vi "auto_test.vi"() -> ()   [LabVIEW 2019]
uses:
  auto_simple_straight.ctl
  <vilib>/Rock Robotics/Network Tables/NT Write Numeric Array.vi
  <vilib>/Rock Robotics/WPI/RobotDrive/WPI_RobotDriveArcadeDrive_Standard(NoSaturation).vi
  <vilib>/Rock Robotics/WPI/Solenoid/WPI_SolenoidValue.ctl
  <vilib>/Rock Robotics/WPI/Solenoid/WPI_SolenoidSetEnum.vi
  <vilib>/Rock Robotics/WPI/ThirdParty/Phoenix-LabVIEW/Motor Controller/Controls/CTRE_Phoenix_MotorControl_ControlMode.ctl
panel:
  out "Output Countdown\nTimer":dbl
  out "Motors and Solenoids On":bool
  out "Auto State":T1
  in  "Abort":bool
  in  "Intake Control":T2 items=["PercentOutput"=0, "Position"=1, "Velocity"=2, "Current"=3, "Follower"=5, "MotionProfile"=6, "MotionMagic"=7, "MotionProfileArc"=10, "Disabled"=15]
  in  "Output Control":T2 items=["PercentOutput"=0, "Position"=1, "Velocity"=2, "Current"=3, "Follower"=5, "MotionProfile"=6, "MotionMagic"=7, "MotionProfileArc"=10, "Disabled"=15]
  in  "Climber Control":T2 items=["PercentOutput"=0, "Position"=1, "Velocity"=2, "Current"=3, "Follower"=5, "MotionProfile"=6, "MotionMagic"=7, "MotionProfileArc"=10, "Disabled"=15]
  in  "Winch Control":T2 items=["PercentOutput"=0, "Position"=1, "Velocity"=2, "Current"=3, "Follower"=5, "MotionProfile"=6, "MotionMagic"=7, "MotionProfileArc"=10, "Disabled"=15]
  in  "Output Control 2":T2 items=["PercentOutput"=0, "Position"=1, "Velocity"=2, "Current"=3, "Follower"=5, "MotionProfile"=6, "MotionMagic"=7, "MotionProfileArc"=10, "Disabled"=15]
  in  "Intake Control":T2 items=["PercentOutput"=0, "Position"=1, "Velocity"=2, "Current"=3, "Follower"=5, "MotionProfile"=6, "MotionMagic"=7, "MotionProfileArc"=10, "Disabled"=15]
  in  "Climber Control":T2 items=["PercentOutput"=0, "Position"=1, "Velocity"=2, "Current"=3, "Follower"=5, "MotionProfile"=6, "MotionMagic"=7, "MotionProfileArc"=10, "Disabled"=15]
  in  "Winch Control":T2 items=["PercentOutput"=0, "Position"=1, "Velocity"=2, "Current"=3, "Follower"=5, "MotionProfile"=6, "MotionMagic"=7, "MotionProfileArc"=10, "Disabled"=15]
  in  "Output Control":T2 items=["PercentOutput"=0, "Position"=1, "Velocity"=2, "Current"=3, "Follower"=5, "MotionProfile"=6, "MotionMagic"=7, "MotionProfileArc"=10, "Disabled"=15]
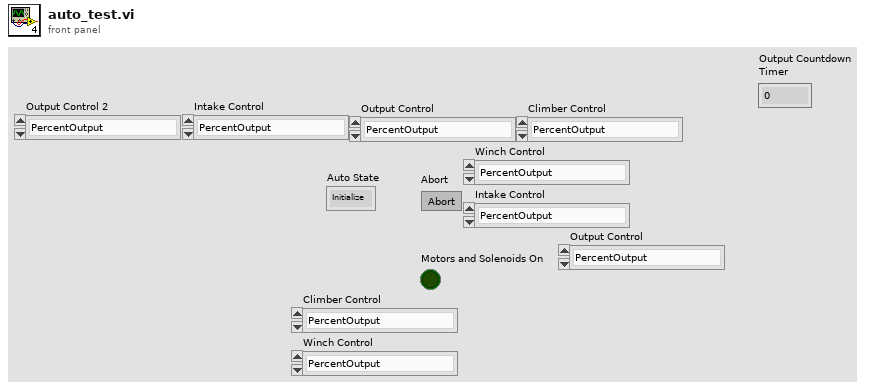
[diagram p1: front panel]
types:
  T1 = typedef "auto_simple_straight.ctl" = enum16{"Initialize", "Ready", "Move Forward", "Start Output Countdown", "Countdown", "Enable Output and Stop Drive", "Abort", "Motors Off"}
  T2 = typedef "CTRE_Phoenix_MotorControl_ControlMode.ctl" = u16
  T3 = typedef "WPI_SolenoidValue.ctl" = enum16{"Off", "On", "Forward", "Reverse"}
  T4 = typedef "WPI_RobotDriveDevRef.ctl" = cluster{"DevStatus":errorcluster, "Motors[]":T5[], "Square Inputs":bool, "Max Output":dbl}
  T5 = typedef "WPI_MotorControlDeviceRef.ctl" = cluster{"DeviceStatus":errorcluster, "Type":T6, "PWM":cluster{"PWM Channel":T7, "DeadBand":T8}, "CAN":cluster{"Device Number":u8, "SetOutput VI Ref":variant, "GetOutput VI Ref":variant, "Enable VI Ref":variant, "Disable VI Ref":variant, "Data":variant}, "Invert":bool, "DIO PWM":cluster{"PWM \"Enable\" Channel":T7, "DIOChannel":T9, "PWM Rate":dbl}}
  T6 = typedef "WPI_MotorControlType.ctl" = enum16{"PWM", "CAN", "DIO PWM"}
  T7 = typedef "FPGA_DIOPWMChannel.ctl" = enum8{"PWM 0", "PWM 1", "PWM 2", "PWM 3", "PWM 4", "PWM 5", "PWM 6", "PWM 7", "PWM 8", "PWM 9", "PWM MXP 0", "PWM MXP 1", "PWM MXP 2", "PWM MXP 3", "PWM MXP 4", "PWM MXP 5", "PWM MXP 6", "PWM MXP 7", "PWM MXP 8", "PWM MXP 9", "Invalid"}
  T8 = typedef "WPI_PWMDeadband.ctl" = cluster{"Name":string, "maxPositivePwm":i32, "minPositivePwm":i32, "centerPwm":i32, "maxNegativePwm":i32, "minNegativePwm":i32, "angularRange":u16}
  T9 = typedef "FPGA_DIOChannel.ctl" = enum8{"DIO 0", "DIO 1", "DIO 2", "DIO 3", "DIO 4", "DIO 5", "DIO 6", "DIO 7", "DIO 8", "DIO 9", "DIO MXP 0", "DIO MXP 1", "DIO MXP 2", "DIO MXP 3", "DIO MXP 4", "DIO MXP 5", "DIO MXP 6", "DIO MXP 7", "DIO MXP 8", "DIO MXP 9", "DIO MXP 10", "DIO MXP 11", "DIO MXP 12", "DIO MXP 13", "DIO MXP 14", "DIO MXP 15", "SPI Port CS1", "SPI Port CS2", "SPI Port CS3", "SPI Port MISO", "SPI Port MOSI", "Invalid"}
  T10 = typedef "WPI_SolenoidDevRef.ctl" = cluster{"DevStatus":errorcluster, "Pneumatics Control Module":u8, "Forward Solenoid Channel":T11, "Reverse Solenoid Channel":T11}
  T11 = typedef "WPI_SolenoidChannel.ctl" = enum8{"Solenoid 0", "Solenoid 1", "Solenoid 2", "Solenoid 3", "Solenoid 4", "Solenoid 5", "Solenoid 6", "Solenoid 7", "Invalid"}
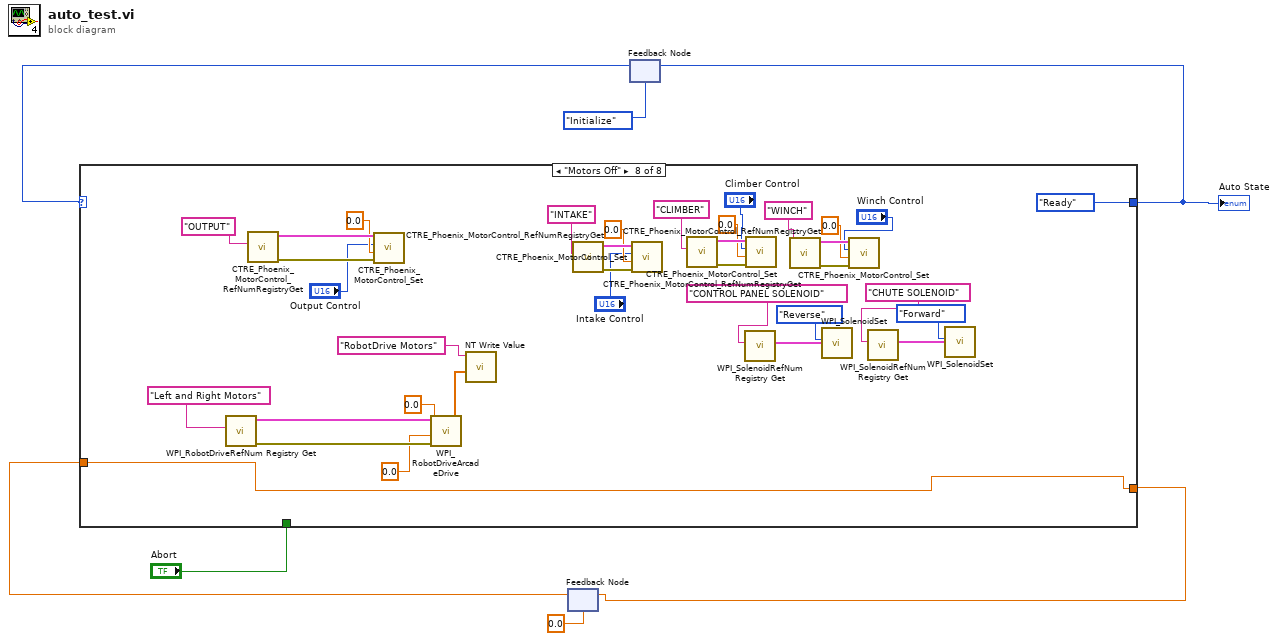
[diagram p0: block diagram]
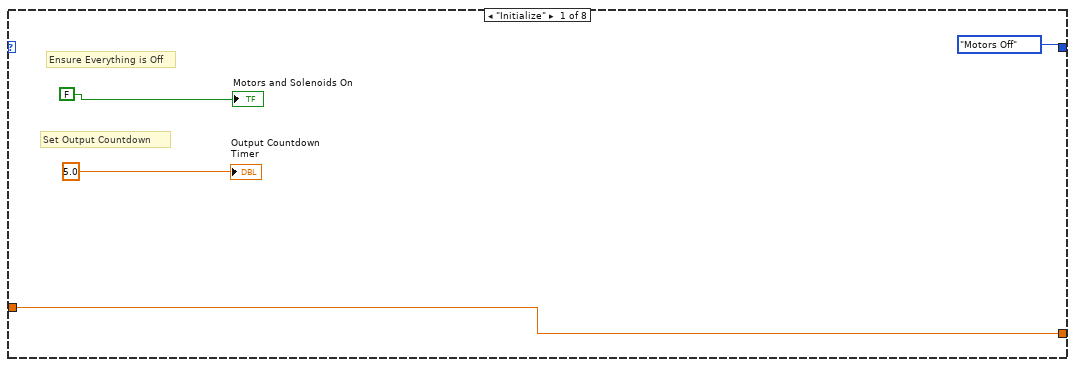
[diagram p2: hidden frame]
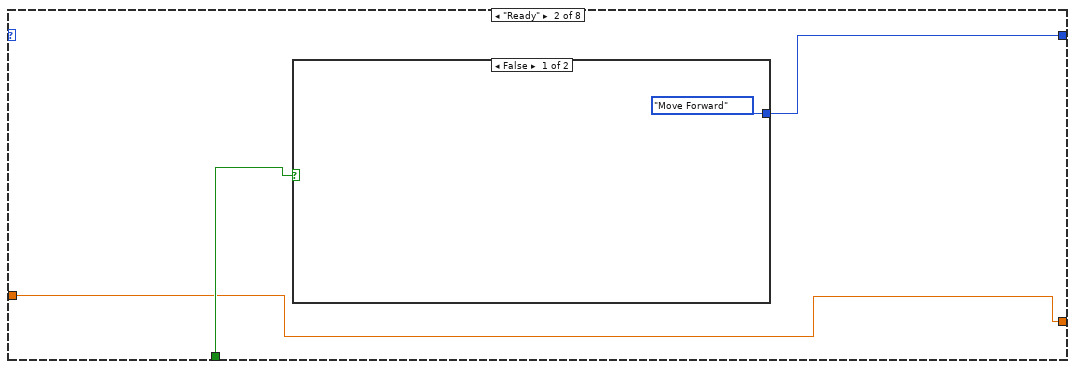
[diagram p3: hidden frame]
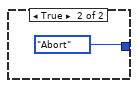
[diagram p4: hidden frame]
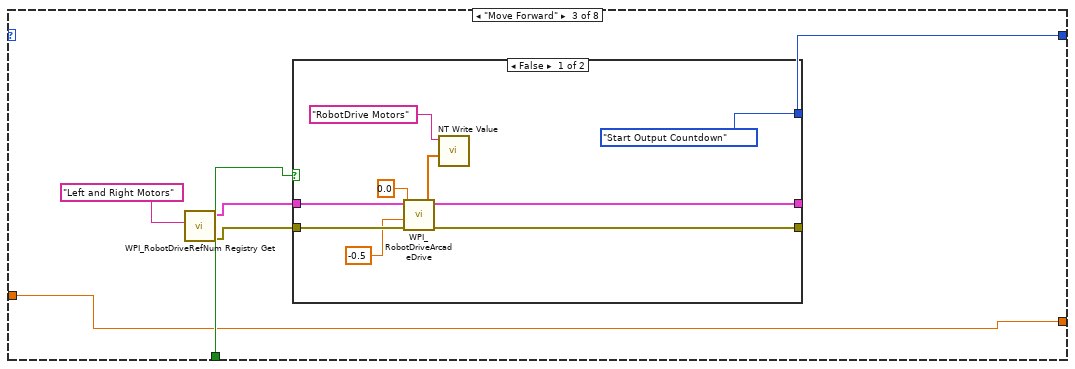
[diagram p5: hidden frame]
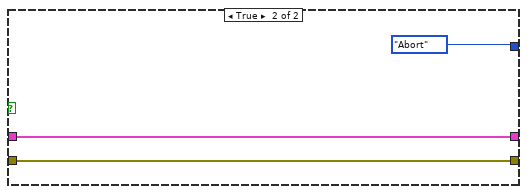
[diagram p6: hidden frame]
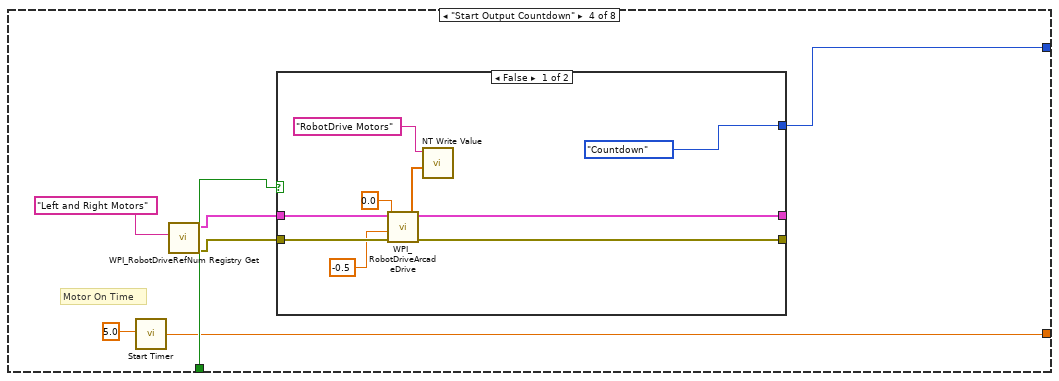
[diagram p7: hidden frame]
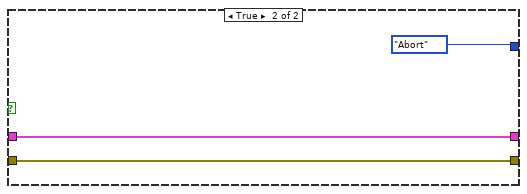
[diagram p8: hidden frame]
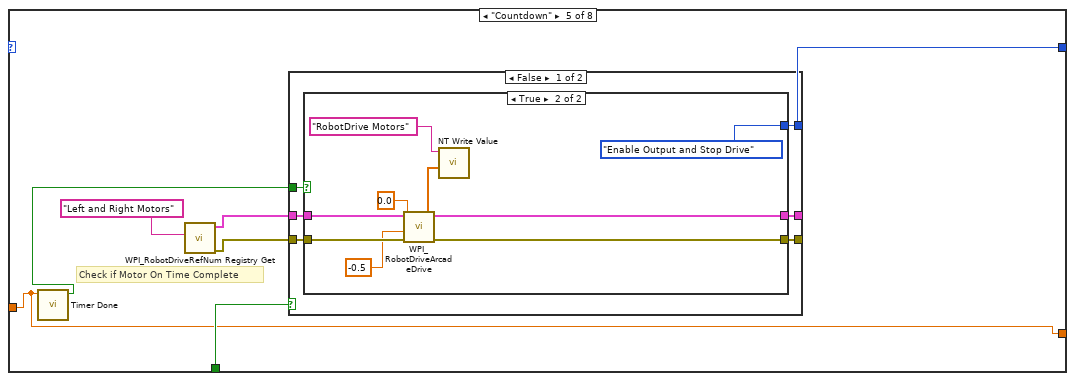
[diagram p9: hidden frame]
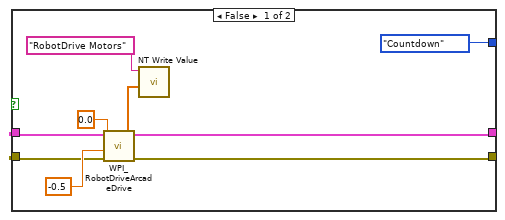
[diagram p10: hidden frame]
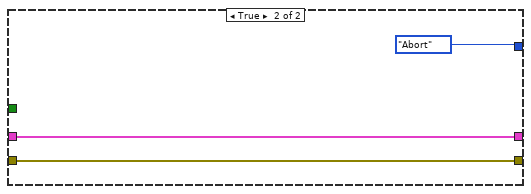
[diagram p11: hidden frame]
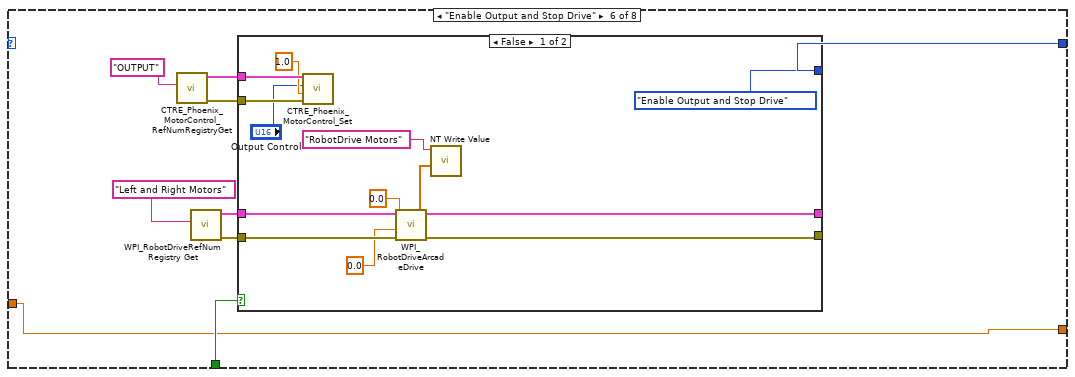
[diagram p12: hidden frame]
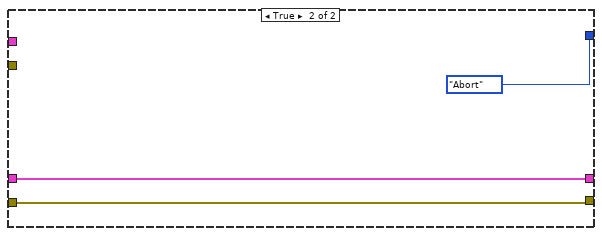
[diagram p13: hidden frame]
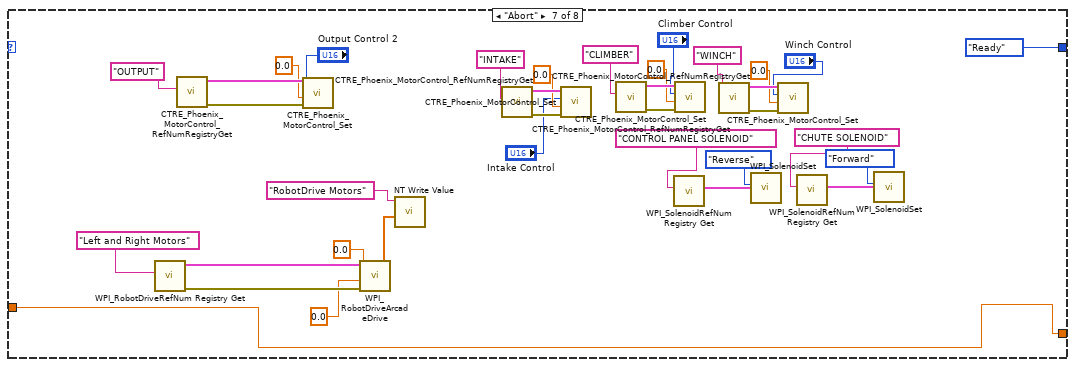
[diagram p14: hidden frame]
diagram:
  n1 = feedback #1(0.0 ("Elapsed Time")) -> (w2:dbl)
  n2 = feedback #2(auto_simple_straight."Initialize" ("Enum")) -> (w4:T1)
  n3 = case shown="\"Motors Off\"" w4 {
    tunnel: "Abort" -> [_ w14 w22 w41 w60 w96 _ _]
    tunnel: [auto_simple_straight."Motors Off" ("Enum") w13 w21 w40 w59 w95 auto_simple_straight."Ready" ("Enum") auto_simple_straight."Ready" ("Enum")] -> w5
    tunnel: [w10 w12 w17 w35 w54 w88 w113 w148] -> w3
    tunnel: w2 -> [w10 w12 w17 _ w54 w88 w113 w148]
    frame "Initialize" {
      # "Set Output Countdown"
      # "Ensure Everything is Off"
      "Motors and Solenoids On" <- FALSE ("Motors and Solenoids On")
      "Output Countdown\nTimer" <- 5.0 ("Countdown\nTimer")
    }
    frame "Ready" {
      n4 = case shown="False" w14 {
        tunnel: [auto_simple_straight."Move Forward" ("Enum") auto_simple_straight."Abort" ("Enum")] -> w13
        frame False {
        }
        frame True {
        }
      }
    }
    frame "Move Forward" {
      n5 = call <vilib>:"WPI_RobotDriveRefNum Registry Get.vi"("refnum name"="Left and Right Motors") -> ("error out"=w18:errorcluster, "RobotDriveDevRef"=w19:T4)  [unwired: 9 in]
      n6 = case shown="False" w22 {
        tunnel: [auto_simple_straight."Start Output Countdown" ("Enum") auto_simple_straight."Abort" ("Enum")] -> w21
        tunnel: w19 -> [w28 w33]
        tunnel: w18 -> [w27 w32]
        tunnel: [w26 w33] -> _
        tunnel: [w23 w32] -> _
        frame False {
          n7 = call-poly <vilib>:"WPI_RobotDriveArcadeDrive.vi"("error in (no error)"=w27, "Y axis value"=-0.5, "X axis value"=0.0, "RobotDriveDevRef"=w28) -> ("error out"=w23:errorcluster, "Motor Values"=w29:dbl[], "RobotDriveDevRef"=w26:T4)  [unwired: 5 out]
          n8 = call-poly <vilib>:"NT Write Value.vi"("Numeric Array"=w29, "Name"="RobotDrive Motors") -> ()  [unwired: 9 in, 1 out]
        }
        frame True {
        }
      }
    }
    frame "Start Output Countdown" {
      # "Motor On Time"
      n9 = call "Start Timer.vi"("Wait\nTime"=5.0 ("Wait\nTime")) -> ("Elapsed Time"=w35:dbl)  [unwired: 10 in]
      n10 = call <vilib>:"WPI_RobotDriveRefNum Registry Get.vi"("refnum name"="Left and Right Motors") -> ("error out"=w37:errorcluster, "RobotDriveDevRef"=w38:T4)  [unwired: 9 in]
      n11 = case shown="False" w41 {
        tunnel: [auto_simple_straight."Countdown" ("Enum") auto_simple_straight."Abort" ("Enum")] -> w40
        tunnel: w38 -> [w47 w52]
        tunnel: w37 -> [w46 w51]
        tunnel: [w45 w52] -> _
        tunnel: [w42 w51] -> _
        frame False {
          n12 = call-poly <vilib>:"WPI_RobotDriveArcadeDrive.vi"("error in (no error)"=w46, "Y axis value"=-0.5, "X axis value"=0.0, "RobotDriveDevRef"=w47) -> ("error out"=w42:errorcluster, "Motor Values"=w48:dbl[], "RobotDriveDevRef"=w45:T4)  [unwired: 5 out]
          n13 = call-poly <vilib>:"NT Write Value.vi"("Numeric Array"=w48, "Name"="RobotDrive Motors") -> ()  [unwired: 9 in, 1 out]
        }
        frame True {
        }
      }
    }
    frame "Countdown" {
      # "Check if Motor On Time Complete"
      n14 = call "Timer Done.vi"("Wait\nTime"=w54) -> ("Timer \nDone?"=w55:bool)  [unwired: 10 in]
      n15 = call <vilib>:"WPI_RobotDriveRefNum Registry Get.vi"("refnum name"="Left and Right Motors") -> ("error out"=w56:errorcluster, "RobotDriveDevRef"=w57:T4)  [unwired: 9 in]
      n16 = case shown="False" w60 {
        tunnel: [w66 auto_simple_straight."Abort" ("Enum")] -> w59
        tunnel: w57 -> [w65 w86]
        tunnel: w56 -> [w64 w85]
        tunnel: [w63 w86] -> _
        tunnel: [w62 w85] -> _
        tunnel: w55 -> [w61 _]
        frame False {
          n17 = case shown="True" w61 {
            tunnel: [auto_simple_straight."Countdown" ("Enum") auto_simple_straight."Enable Output and Stop Drive" ("Enum")] -> w66
            tunnel: w65 -> [w71 w81]
            tunnel: w64 -> [w70 w80]
            tunnel: [w69 w79] -> w63
            tunnel: [w68 w76] -> w62
            frame False {
              n18 = call-poly <vilib>:"WPI_RobotDriveArcadeDrive.vi"("error in (no error)"=w70, "Y axis value"=-0.5, "X axis value"=0.0, "RobotDriveDevRef"=w71) -> ("error out"=w68:errorcluster, "Motor Values"=w74:dbl[], "RobotDriveDevRef"=w69:T4)  [unwired: 5 out]
              n19 = call-poly <vilib>:"NT Write Value.vi"("Numeric Array"=w74, "Name"="RobotDrive Motors") -> ()  [unwired: 9 in, 1 out]
            }
            frame True {
              n20 = call-poly <vilib>:"WPI_RobotDriveArcadeDrive.vi"("error in (no error)"=w80, "Y axis value"=-0.5, "X axis value"=0.0, "RobotDriveDevRef"=w81) -> ("error out"=w76:errorcluster, "Motor Values"=w82:dbl[], "RobotDriveDevRef"=w79:T4)  [unwired: 5 out]
              n21 = call-poly <vilib>:"NT Write Value.vi"("Numeric Array"=w82, "Name"="RobotDrive Motors") -> ()  [unwired: 9 in, 1 out]
            }
          }
        }
        frame True {
        }
      }
    }
    frame "Enable Output and Stop Drive" {
      n22 = call <vilib>:"CTRE_Phoenix_MotorControl_RefNumRegistryGet.vi"("refnum name"="OUTPUT") -> ("error out"=w91:errorcluster, "PhoenixMotorControlDevRef"=w90:T5)  [unwired: 9 in]
      n23 = call <vilib>:"WPI_RobotDriveRefNum Registry Get.vi"("refnum name"="Left and Right Motors") -> ("error out"=w92:errorcluster, "RobotDriveDevRef"=w93:T4)  [unwired: 9 in]
      n24 = case shown="False" w96 {
        tunnel: [auto_simple_straight."Enable Output and Stop Drive" ("Enum") auto_simple_straight."Abort" ("Enum")] -> w95
        tunnel: w93 -> [w108 w111]
        tunnel: w92 -> [w107 w110]
        tunnel: [w106 w111] -> _
        tunnel: [w105 w110] -> _
        tunnel: w91 -> [w100 _]
        tunnel: w90 -> [w99 _]
        frame False {
          n25 = call <vilib>:"CTRE_Phoenix_MotorControl_Set.vi"("error in (no error)"=w100, "Output"=1.0, "Control Mode"="Output Control", "PhoenixMotorControlDevRef"=w99) -> ()  [unwired: 6 in, 2 out]
          n26 = call-poly <vilib>:"WPI_RobotDriveArcadeDrive.vi"("error in (no error)"=w107, "Y axis value"=0.0, "X axis value"=0.0, "RobotDriveDevRef"=w108) -> ("error out"=w105:errorcluster, "Motor Values"=w103:dbl[], "RobotDriveDevRef"=w106:T4)  [unwired: 5 out]
          n27 = call-poly <vilib>:"NT Write Value.vi"("Numeric Array"=w103, "Name"="RobotDrive Motors") -> ()  [unwired: 9 in, 1 out]
        }
        frame True {
        }
      }
    }
    frame "Abort" {
      n28 = call <vilib>:"WPI_RobotDriveRefNum Registry Get.vi"("refnum name"="Left and Right Motors") -> ("error out"=w144:errorcluster, "RobotDriveDevRef"=w145:T4)  [unwired: 9 in]
      n29 = call <vilib>:"CTRE_Phoenix_MotorControl_RefNumRegistryGet.vi"("refnum name"="OUTPUT") -> ("error out"=w143:errorcluster, "PhoenixMotorControlDevRef"=w142:T5)  [unwired: 9 in]
      n30 = call <vilib>:"CTRE_Phoenix_MotorControl_Set.vi"("error in (no error)"=w143, "Output"=0.0, "Control Mode"="Output Control 2", "PhoenixMotorControlDevRef"=w142) -> ()  [unwired: 6 in, 2 out]
      n31 = call-poly <vilib>:"WPI_RobotDriveArcadeDrive.vi"("error in (no error)"=w144, "Y axis value"=0.0, "X axis value"=0.0, "RobotDriveDevRef"=w145) -> ("Motor Values"=w139:dbl[])  [unwired: 7 out]
      n32 = call-poly <vilib>:"NT Write Value.vi"("Numeric Array"=w139, "Name"="RobotDrive Motors") -> ()  [unwired: 9 in, 1 out]
      n33 = call <vilib>:"CTRE_Phoenix_MotorControl_RefNumRegistryGet.vi"("refnum name"="INTAKE") -> ("error out"=w133:errorcluster, "PhoenixMotorControlDevRef"=w134:T5)  [unwired: 9 in]
      n34 = call <vilib>:"CTRE_Phoenix_MotorControl_Set.vi"("error in (no error)"=w133, "Output"=0.0, "Control Mode"="Intake Control", "PhoenixMotorControlDevRef"=w134) -> ()  [unwired: 6 in, 2 out]
      n35 = call <vilib>:"CTRE_Phoenix_MotorControl_RefNumRegistryGet.vi"("refnum name"="CLIMBER") -> ("error out"=w130:errorcluster, "PhoenixMotorControlDevRef"=w131:T5)  [unwired: 9 in]
      n36 = call <vilib>:"WPI_SolenoidRefNum Registry Get.vi"("refnum name"="CONTROL PANEL SOLENOID") -> ("SolenoidDevRef"=w123:T10)  [unwired: 9 in, 1 out]
      n37 = call <vilib>:"CTRE_Phoenix_MotorControl_Set.vi"("error in (no error)"=w130, "Output"=0.0, "Control Mode"="Climber Control", "PhoenixMotorControlDevRef"=w131) -> ()  [unwired: 6 in, 2 out]
      n38 = call <vilib>:"CTRE_Phoenix_MotorControl_RefNumRegistryGet.vi"("refnum name"="WINCH") -> ("error out"=w126:errorcluster, "PhoenixMotorControlDevRef"=w127:T5)  [unwired: 9 in]
      n39 = call-poly <vilib>:"WPI_SolenoidSet.vi"("Value"=WPI_SolenoidValue."Reverse", "SolenoidDevRef"=w123) -> ()  [unwired: 8 in, 2 out]
      n40 = call <vilib>:"CTRE_Phoenix_MotorControl_Set.vi"("error in (no error)"=w126, "Output"=0.0, "Control Mode"="Winch Control", "PhoenixMotorControlDevRef"=w127) -> ()  [unwired: 6 in, 2 out]
      n41 = call <vilib>:"WPI_SolenoidRefNum Registry Get.vi"("refnum name"="CHUTE SOLENOID") -> ("SolenoidDevRef"=w121:T10)  [unwired: 9 in, 1 out]
      n42 = call-poly <vilib>:"WPI_SolenoidSet.vi"("Value"=WPI_SolenoidValue."Forward", "SolenoidDevRef"=w121) -> ()  [unwired: 8 in, 2 out]
    }
    frame "Motors Off" {
      n43 = call <vilib>:"WPI_RobotDriveRefNum Registry Get.vi"("refnum name"="Left and Right Motors") -> ("error out"=w179:errorcluster, "RobotDriveDevRef"=w180:T4)  [unwired: 9 in]
      n44 = call <vilib>:"CTRE_Phoenix_MotorControl_RefNumRegistryGet.vi"("refnum name"="OUTPUT") -> ("error out"=w178:errorcluster, "PhoenixMotorControlDevRef"=w177:T5)  [unwired: 9 in]
      n45 = call <vilib>:"CTRE_Phoenix_MotorControl_Set.vi"("error in (no error)"=w178, "Output"=0.0, "Control Mode"="Output Control", "PhoenixMotorControlDevRef"=w177) -> ()  [unwired: 6 in, 2 out]
      n46 = call-poly <vilib>:"WPI_RobotDriveArcadeDrive.vi"("error in (no error)"=w179, "Y axis value"=0.0, "X axis value"=0.0, "RobotDriveDevRef"=w180) -> ("Motor Values"=w174:dbl[])  [unwired: 7 out]
      n47 = call-poly <vilib>:"NT Write Value.vi"("Numeric Array"=w174, "Name"="RobotDrive Motors") -> ()  [unwired: 9 in, 1 out]
      n48 = call <vilib>:"CTRE_Phoenix_MotorControl_RefNumRegistryGet.vi"("refnum name"="INTAKE") -> ("error out"=w168:errorcluster, "PhoenixMotorControlDevRef"=w169:T5)  [unwired: 9 in]
      n49 = call <vilib>:"CTRE_Phoenix_MotorControl_Set.vi"("error in (no error)"=w168, "Output"=0.0, "Control Mode"="Intake Control", "PhoenixMotorControlDevRef"=w169) -> ()  [unwired: 6 in, 2 out]
      n50 = call <vilib>:"CTRE_Phoenix_MotorControl_RefNumRegistryGet.vi"("refnum name"="CLIMBER") -> ("error out"=w165:errorcluster, "PhoenixMotorControlDevRef"=w166:T5)  [unwired: 9 in]
      n51 = call <vilib>:"WPI_SolenoidRefNum Registry Get.vi"("refnum name"="CONTROL PANEL SOLENOID") -> ("SolenoidDevRef"=w158:T10)  [unwired: 9 in, 1 out]
      n52 = call <vilib>:"CTRE_Phoenix_MotorControl_Set.vi"("error in (no error)"=w165, "Output"=0.0, "Control Mode"="Climber Control", "PhoenixMotorControlDevRef"=w166) -> ()  [unwired: 6 in, 2 out]
      n53 = call <vilib>:"CTRE_Phoenix_MotorControl_RefNumRegistryGet.vi"("refnum name"="WINCH") -> ("error out"=w161:errorcluster, "PhoenixMotorControlDevRef"=w162:T5)  [unwired: 9 in]
      n54 = call-poly <vilib>:"WPI_SolenoidSet.vi"("Value"=WPI_SolenoidValue."Reverse", "SolenoidDevRef"=w158) -> ()  [unwired: 8 in, 2 out]
      n55 = call <vilib>:"CTRE_Phoenix_MotorControl_Set.vi"("error in (no error)"=w161, "Output"=0.0, "Control Mode"="Winch Control", "PhoenixMotorControlDevRef"=w162) -> ()  [unwired: 6 in, 2 out]
      n56 = call <vilib>:"WPI_SolenoidRefNum Registry Get.vi"("refnum name"="CHUTE SOLENOID") -> ("SolenoidDevRef"=w156:T10)  [unwired: 9 in, 1 out]
      n57 = call-poly <vilib>:"WPI_SolenoidSet.vi"("Value"=WPI_SolenoidValue."Forward", "SolenoidDevRef"=w156) -> ()  [unwired: 8 in, 2 out]
    }
  }
  "Auto State" <- w5
  n58 = feedback-in #1(w3) -> ()
  n59 = feedback-in #2(w5) -> ()
